vi "get_average_roi_spectrum.vi"(1 "ROI":T1, 3 "CUBE":sgl[][][](array[numeric])) -> (0 "SPECTRA":dbl[][](array[numeric]))   [LabVIEW 2018]
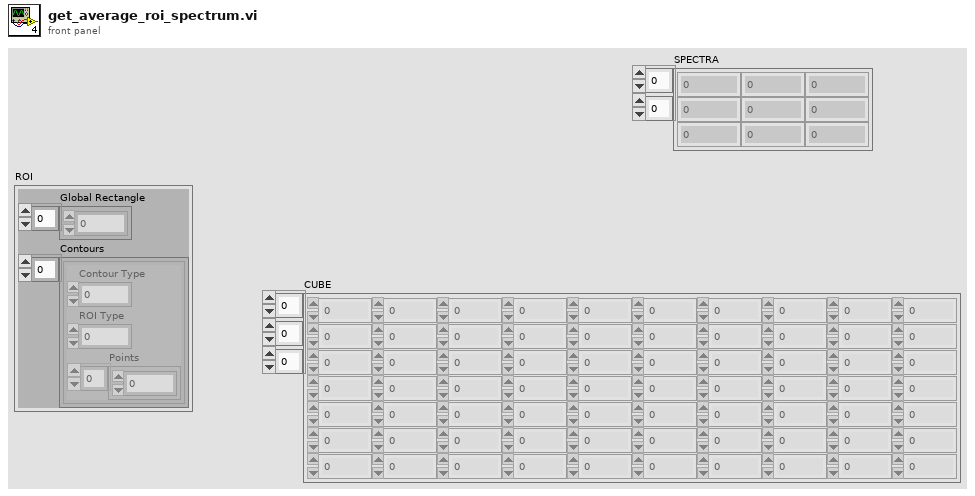
[diagram p1: front panel]
types:
  T1 = cluster{"Global Rectangle":i32[], "Contours":cluster{"Contour Type":u32, "ROI Type":u32, "Points":i32[]}[]}
  T2 = cluster{"Contour Type":u32, "ROI Type":u32, "Points":i32[]}[]
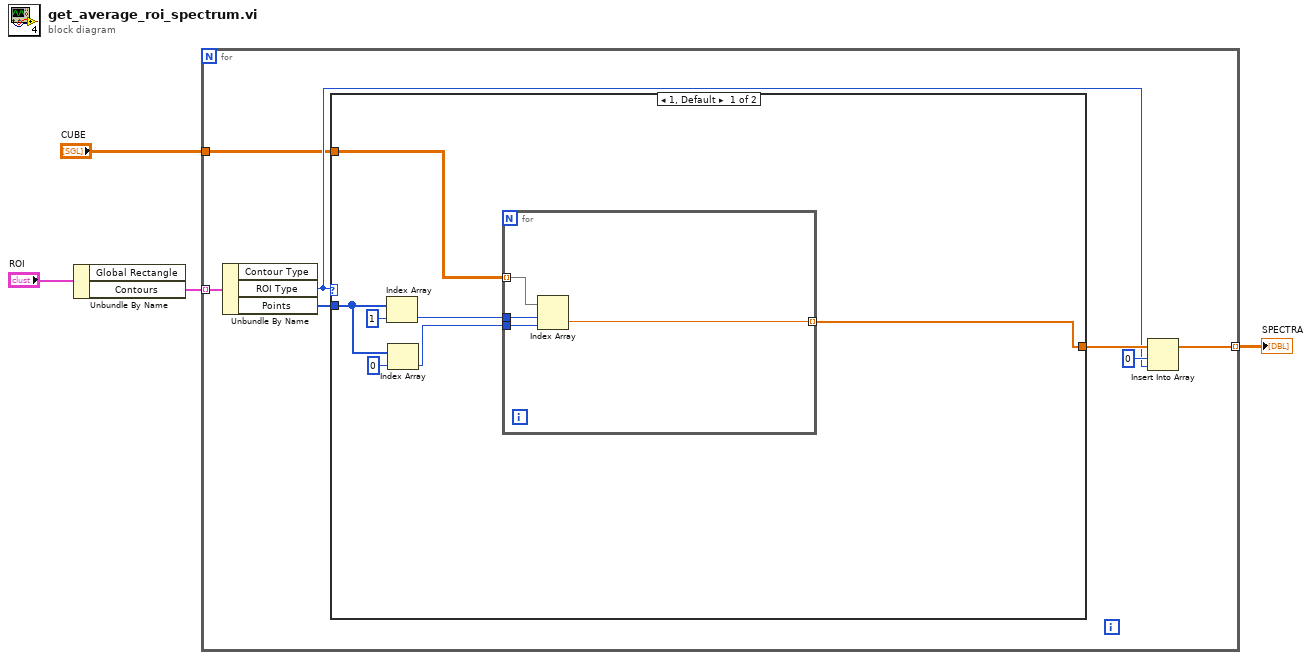
[diagram p0: block diagram]
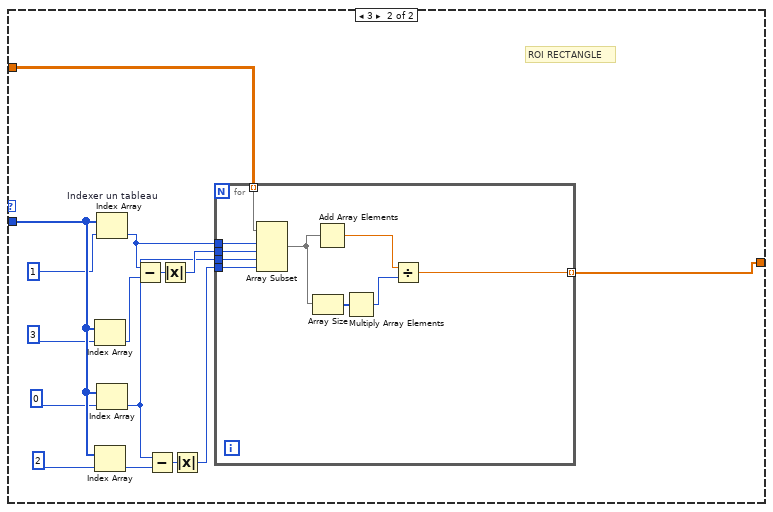
[diagram p2: hidden frame]
diagram:
  n1 = Unbundle By Name("ROI") -> ("Contours"=w3:T2)  [unwired: 1 out]
  n2 = for {
    tunnel: w3 -> [w11] mode=indexing
    tunnel: [w6] -> w2 mode=indexing
    tunnel: "CUBE" -> [w5]
    n3 = Unbundle By Name(w11) -> ("ROI Type"=w7:u32, "Points"=w10:i32[])  [unwired: 1 out]
    n4 = case shown="1, Default" w7 {
      tunnel: w10 -> [w18 w37]
      tunnel: [w12 w31] -> w9
      tunnel: w5 -> [w15 w32]
      frame 1, Default {
        n5 = Index Array(array=w18, index=1 ("indice")) -> (element=w14:i32)
        n6 = Index Array(array=w18, index=0 ("indice")) -> (element=w13:i32)
        n7 = for {
          tunnel: w15 -> [w22] mode=indexing
          tunnel: w14 -> [w21]
          tunnel: w13 -> [w20]
          tunnel: [w19] -> w12 mode=indexing
          n8 = Index Array(array=w22, index (row)=w21, index (col)=w20) -> (element=w19:sgl)
        }
      }
      frame 3 {
        # "ROI RECTANGLE"
        n9 = Index Array(array=w37, index=3 ("indice")) -> (element=w27:i32)
        n10 = Index Array(array=w37, index=2 ("indice")) -> (element=w29:i32)
        n11 = Index Array "Indexer un tableau"(array=w37, index=1 ("indice")) -> (element=w26:i32)
        n12 = Index Array(array=w37, index=0 ("indice")) -> (element=w24:i32)
        n13 = Subtract(x=w26, y=w27) -> (x-y=w28:i32)
        n14 = Subtract(x=w24, y=w29) -> (x-y=w30:i32)
        n15 = Absolute Value(x=w28) -> (abs(x)=w25:i32)
        n16 = Absolute Value(x=w30) -> (abs(x)=w23:i32)
        n17 = for {
          tunnel: w32 -> [w47] mode=indexing
          tunnel: [w42] -> w31 mode=indexing
          tunnel: w26 -> [w41]
          tunnel: w25 -> [w40]
          tunnel: w24 -> [w39]
          tunnel: w23 -> [w38]
          n18 = Array Subset(array=w47, index (row)=w41, length (row)=w40, index (col)=w39, length (col)=w38) -> (w45:sgl[][])
          n19 = Array Size(array=w45) -> (size(s)=w46:i32[])
          n20 = Add Array Elements(numeric array=w45) -> (sum=w44:sgl)
          n21 = Multiply Array Elements(1:w46) -> (0:w43:i32)
          n22 = Divide(x=w44, y=w43) -> (x/y=w42:sgl)
        }
      }
    }
    n23 = Insert Into Array(array=w9, index=0 ("indice"), new element=w7) -> (w6:sgl[])
  }
  "SPECTRA" <- w2
